vi "Scalar SV Count - String Type Array.vi"(8 "Error In":errorcluster, 10 "Initial number":i32, 11 "Type array":string[](array[string])) -> (0 "Error Out":errorcluster, 2 "Number of scalar SV":i32)   [LabVIEW 2014]
doc: "This VI counts the number of scalar shared variables."
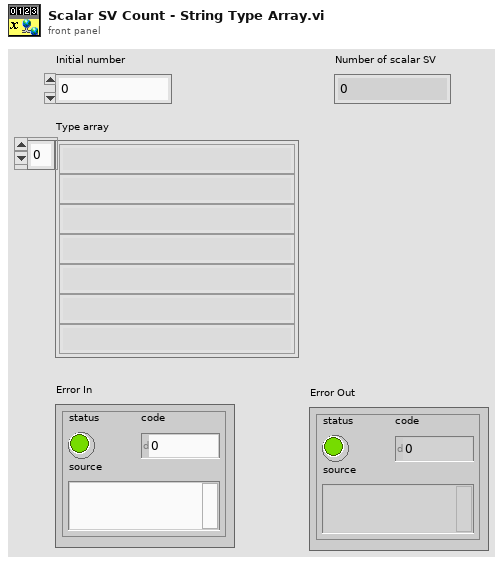
[diagram p1: front panel]
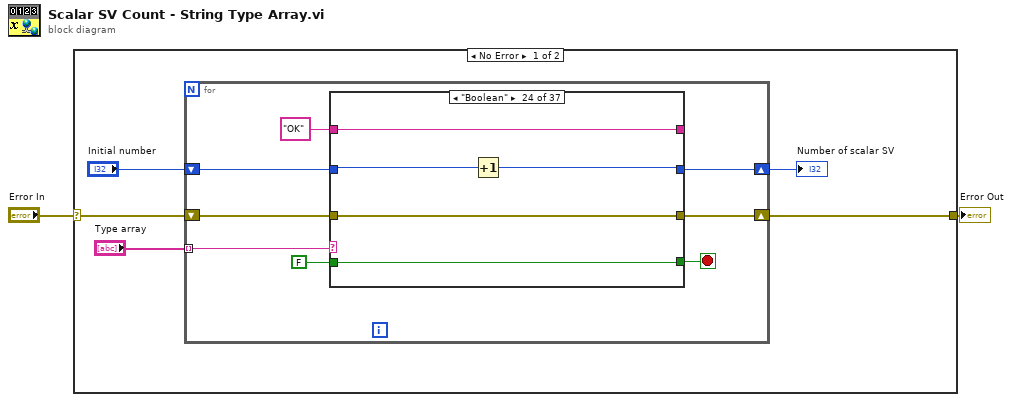
[diagram p0: block diagram]
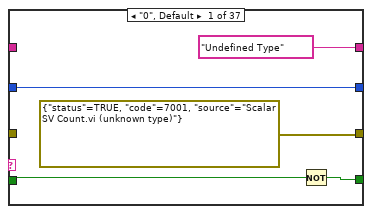
[diagram p2: hidden frame]
diagram:
  n1 = case shown="No Error" "Error In" {
    selector: "Error In" -> [w7 w179]
    tunnel: [w6 w179] -> w1
    frame No Error {
      n2 = for {
        shift-right: [w14] -> w6
        shift-left: w7 -> [w15]
        tunnel: "Type array" -> [w10] mode=indexing
        shift-right: [w8] -> w3
        shift-left: "Initial number" -> [w9]
        stop <- w11 stop-if-true
        n3 = case shown="\"Boolean\"" w10 {
          tunnel: w15 -> [_ w21 w25 w29 w33 w37 w41 w45 w49 w53 w57 w61 w65 w69 w73 w77 w81 w85 w89 w93 w97 w101 w105 w111 w116 w121 w126 w131 w136 w141 w146 w152 w156 w161 w166 w171 w176]
          tunnel: [errorcluster {"status"=TRUE, "code"=7001, "source"="Scalar SV Count.vi (unknown type)"} ("error constant") w21 w25 w29 w33 w37 w41 w45 w49 w53 w57 w61 w65 w69 w73 w77 w81 w85 w89 w93 w97 w101 w105 w111 w116 w121 w126 w131 w136 w141 w146 w152 w156 w161 w166 w171 w176] -> w14
          tunnel: ["Undefined Type" w24 w28 w32 w36 w40 w44 w48 w52 w56 w60 w64 w68 w72 w76 w80 w84 w88 w92 w96 w100 w104 w108 w113 w118 w123 w128 w133 w138 w143 w148 w153 w158 w163 w168 w173 w178] -> _
          tunnel: "OK" -> [_ w24 w28 w32 w36 w40 w44 w48 w52 w56 w60 w64 w68 w72 w76 w80 w84 w88 w92 w96 w100 w104 w108 w113 w118 w123 w128 w133 w138 w143 w148 w153 w158 w163 w168 w173 w178]
          tunnel: FALSE -> [w19 w23 w27 w31 w35 w39 w43 w47 w51 w55 w59 w63 w67 w71 w75 w79 w83 w87 w91 w95 w99 w103 w107 w112 w117 w122 w127 w132 w137 w142 w147 w149 w157 w162 w167 w172 w177]
          tunnel: [w18 w23 w27 w31 w35 w39 w43 w47 w51 w55 w59 w63 w67 w71 w75 w79 w83 w87 w91 w95 w99 w103 w107 w112 w117 w122 w127 w132 w137 w142 w147 w149 w157 w162 w167 w172 w177] -> w11
          tunnel: w9 -> [w16 w22 w26 w30 w34 w38 w42 w46 w50 w54 w58 w62 w66 w70 w74 w78 w82 w86 w90 w94 w98 w102 w106 w110 w115 w120 w125 w130 w135 w140 w145 w151 w155 w160 w165 w170 w175]
          tunnel: [w16 w22 w26 w30 w34 w38 w42 w46 w50 w54 w58 w62 w66 w70 w74 w78 w82 w86 w90 w94 w98 w102 w106 w109 w114 w119 w124 w129 w134 w139 w144 w150 w154 w159 w164 w169 w174] -> w8
          frame "0", Default {
            n4 = Not(x=w19) -> (.not. x?=w18:bool)
          }
          frame "1D array of Boolean" {
          }
          frame "1D array of Double" {
          }
          frame "1D array of Int16" {
          }
          frame "1D array of Int32" {
          }
          frame "1D array of Int64" {
          }
          frame "1D array of Int8" {
          }
          frame "1D array of Single-precision" {
          }
          frame "1D array of UInt16" {
          }
          frame "1D array of UInt32" {
          }
          frame "1D array of UInt64" {
          }
          frame "1D array of UInt8" {
          }
          frame "2D array of Boolean" {
          }
          frame "2D array of Double" {
          }
          frame "2D array of Int16" {
          }
          frame "2D array of Int32" {
          }
          frame "2D array of Int64" {
          }
          frame "2D array of Int8" {
          }
          frame "2D array of Single-precision" {
          }
          frame "2D array of UInt16" {
          }
          frame "2D array of UInt32" {
          }
          frame "2D array of UInt64" {
          }
          frame "2D array of UInt8" {
          }
          frame "Boolean" {
            n5 = Increment(x=w110) -> (x+1=w109:i32)
          }
          frame "String" {
            n6 = Increment(x=w115) -> (x+1=w114:i32)
          }
          frame "Double" {
            n7 = Increment(x=w120) -> (x+1=w119:i32)
          }
          frame "Fixed Point - signed" {
            n8 = Increment(x=w125) -> (x+1=w124:i32)
          }
          frame "Fixed Point - unsigned" {
            n9 = Increment(x=w130) -> (x+1=w129:i32)
          }
          frame "Int16" {
            n10 = Increment(x=w135) -> (x+1=w134:i32)
          }
          frame "Int32" {
            n11 = Increment(x=w140) -> (x+1=w139:i32)
          }
          frame "Int64" {
            n12 = Increment(x=w145) -> (x+1=w144:i32)
          }
          frame "Int8" {
            n13 = Increment(x=w151) -> (x+1=w150:i32)
          }
          frame "Single-precision" {
            n14 = Increment(x=w155) -> (x+1=w154:i32)
          }
          frame "UInt16" {
            n15 = Increment(x=w160) -> (x+1=w159:i32)
          }
          frame "UInt32" {
            n16 = Increment(x=w165) -> (x+1=w164:i32)
          }
          frame "UInt64" {
            n17 = Increment(x=w170) -> (x+1=w169:i32)
          }
          frame "UInt8" {
            n18 = Increment(x=w175) -> (x+1=w174:i32)
          }
        }
      }
      "Number of scalar SV" <- w3
    }
    frame Error {
    }
  }
  "Error Out" <- w1
